vi "Plotting.vi"(0 "Display Inner Loop":bool, 5 "Display Outer Loop":bool, 7 "Inner Loop State in":T3, 9 "Outer Loop State in":T1 {"Phi Setpoint" format="%#_13g"}, 11 "error in (no error)":errorcluster) -> (4 "U plot":cluster{"U saturated":sgl, "U":dbl}, 8 "Theta (Deg)":dbl, 10 "Theta Ref Plot":T2, 15 "error out":errorcluster)   [LabVIEW 2014]
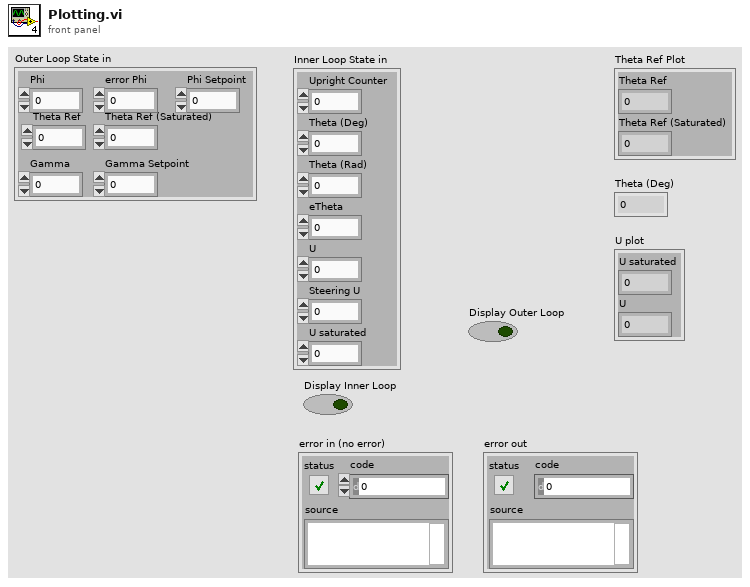
[diagram p1: front panel]
types:
  T1 = cluster{"Phi":dbl, "error Phi":dbl, "Gamma":dbl, "Theta Ref":dbl, "Theta Ref (Saturated)":sgl, "Gamma Setpoint":dbl, "Phi Setpoint":dbl}
  T2 = cluster{"Theta Ref":dbl, "Theta Ref (Saturated)":sgl}
  T3 = cluster{"Upright Counter":dbl, "Theta (Deg)":dbl, "Theta (Rad)":dbl, "eTheta":dbl, "U":dbl, "Steering U":dbl, "U saturated":sgl}
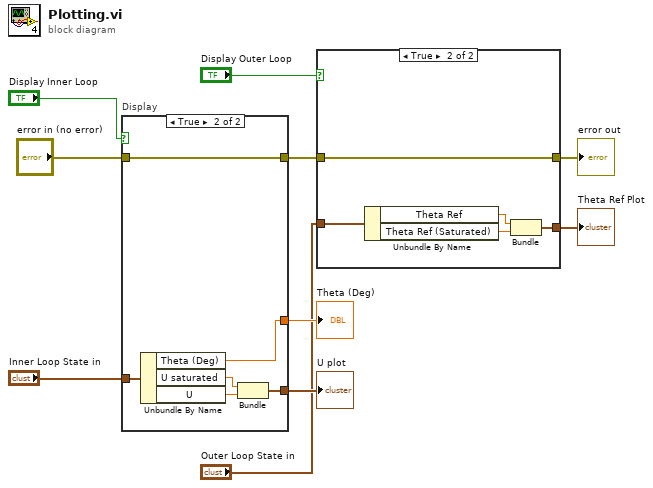
[diagram p0: block diagram]
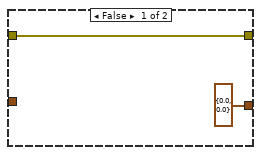
[diagram p2: hidden frame]
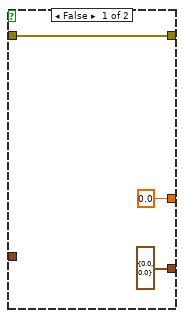
[diagram p3: hidden frame]
diagram:
  n1 = case "Display" shown="True" "Display Inner Loop" {
    tunnel: "error in (no error)" -> [w13 w17]
    tunnel: [w13 w17] -> w5
    tunnel: [cluster{"U saturated":sgl, "U":dbl} {"U saturated"=0.0, "U"=0.0} w16] -> w7
    tunnel: "Inner Loop State in" -> [_ w15]
    tunnel: [0.0 ("Theta (Deg)") w14] -> w10
    frame False {
    }
    frame True {
      n2 = Unbundle By Name(w15) -> ("Theta (Deg)"=w14:dbl, "U saturated"=w19:sgl, "U"=w18:dbl)
      n3 = Bundle("U saturated"=w19, "U"=w18) -> (w16:cluster{"U saturated":sgl, "U":dbl})  [unwired: 1 in]
    }
  }
  "Theta (Deg)" <- w10
  "U plot" <- w7
  n4 = case shown="True" "Display Outer Loop" {
    tunnel: w5 -> [w21 w24]
    tunnel: [w21 w24] -> w6
    tunnel: [T2 {"Theta Ref"=0.0, "Theta Ref (Saturated)"=0.0} w23] -> w8
    tunnel: "Outer Loop State in" -> [_ w22]
    frame False {
    }
    frame True {
      n5 = Unbundle By Name(w22) -> ("Theta Ref"=w26:dbl, "Theta Ref (Saturated)"=w25:sgl)
      n6 = Bundle("Theta Ref"=w26, "Theta Ref (Saturated)"=w25) -> (w23:T2)  [unwired: 1 in]
    }
  }
  "Theta Ref Plot" <- w8
  "error out" <- w6
